vi "Rename State.vi"(8 "error in":errorcluster, 9 "new state":string, 10 "state":string, 11 "routing channel in":T1 format="%.0x") -> (0 "error out":errorcluster, 3 "routing channel out":T1=18446744073709551615 format="%.0x")   [LabVIEW 2020, in "Routing and Faulting Scripting.lvlib"]
doc: "Changes the name of an existing state."
uses:
  Routing and Faulting Scripting.lvlib
  <vilib>/NI VeriStand/Custom Device API/Custom Device Item Ref.ctl
  <vilib>/NI VeriStand/Custom Device API/Custom Device API.lvlib
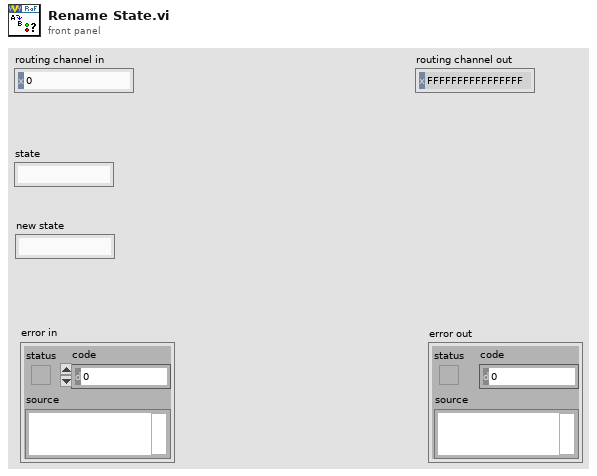
[diagram p1: front panel]
types:
  T1 = typedef "Custom Device API.lvlib/Custom Device Item Ref.ctl" = u64
  T2 = typedef "Routing and Faulting Shared.lvlib/Channel States.ctl" = T3[]
  T3 = typedef "Routing and Faulting Shared.lvlib/Routing State.ctl" = cluster{"Name":string, "Description":string, "Value":i32, "Connection List":T4[]}
  T4 = typedef "Routing and Faulting Shared.lvlib/Connection.ctl" = cluster{"Module":string, "Source":string, "Destination":string}
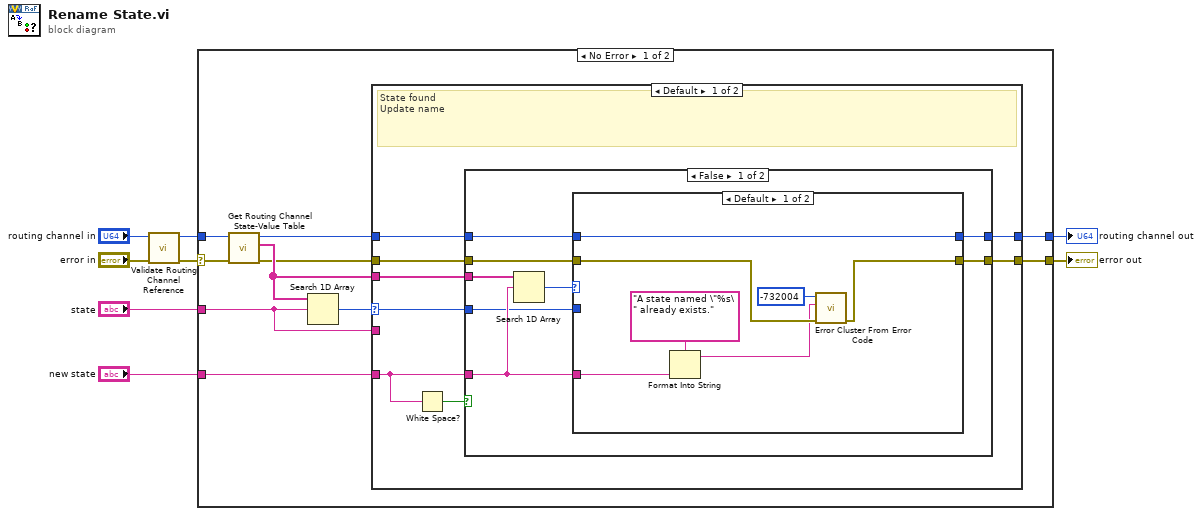
[diagram p0: block diagram]
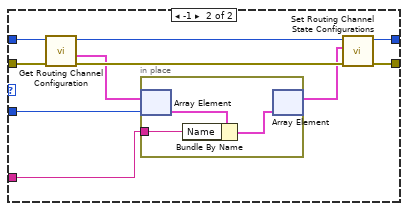
[diagram p2: hidden frame]
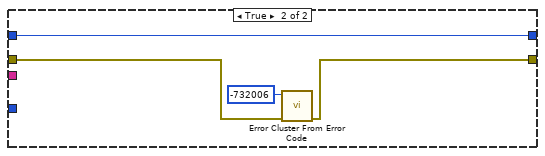
[diagram p3: hidden frame]
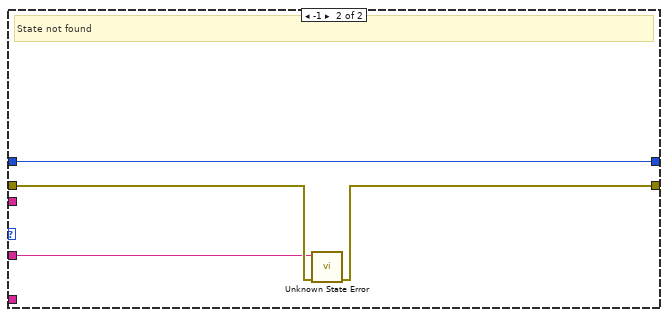
[diagram p4: hidden frame]
diagram:
  n1 = call "Validate Routing Channel Reference.vi"("error in"="error in", "routing channel in"="routing channel in") -> ("error out"=w3:errorcluster, "routing channel out"=w1:T1)  [unwired: 8 in]
  n2 = case shown="No Error" w3 {
    selector: w3 -> [w17 w64]
    tunnel: [w14 w64] -> w5
    tunnel: w1 -> [w18 w63]
    tunnel: [w15 w63] -> w7
    tunnel: "state" -> [w10 _]
    tunnel: "new state" -> [w12 _]
    frame No Error {
      n3 = call "Get Routing Channel State-Value Table.vi"("error in"=w17, "routing channel in"=w18) -> ("error out"=w9:errorcluster, "state names"=w13:string[], "routing channel out"=w16:T1)  [unwired: 6 in, 1 out]
      n4 = Search 1D Array(1D array=w13, element=w10) -> (index of element=w11:i32)  [unwired: 1 in]
      n5 = case shown="Default" w11 {
        selector: w11 -> [w21 _]
        tunnel: w16 -> [w26 w60]
        tunnel: w9 -> [w25 w62]
        tunnel: [w22 w60] -> w15
        tunnel: [w23 w61] -> w14
        tunnel: w12 -> [w20 _]
        tunnel: w13 -> [w24 _]
        tunnel: w10 -> [_ w59]
        frame Default {
          # "State found\nUpdate name"
          n6 = White Space?(1:w20) -> (0:w19:bool)
          n7 = case shown="False" w19 {
            tunnel: w26 -> [w34 w57]
            tunnel: w25 -> [w33 w56]
            tunnel: w24 -> [w32 _]
            tunnel: w20 -> [w31 _]
            tunnel: [w30 w55] -> w23
            tunnel: [w28 w57] -> w22
            tunnel: w21 -> [w27 _]
            frame False {
              n8 = Search 1D Array(1D array=w32, element=w31) -> (index of element=w29:i32)  [unwired: 1 in]
              n9 = case shown="Default" w29 {
                tunnel: w34 -> [w39 w49]
                tunnel: w33 -> [w40 w42]
                tunnel: w31 -> [w36 w48]
                tunnel: [w38 w43] -> w30
                tunnel: [w39 w44] -> w28
                tunnel: w27 -> [_ w47]
                frame Default {
                  n10 = Format Into String(format string="A state named \"%s\" already exists." ("error message (\"\")"), w36) -> (resulting string=w35:string)  [unwired: 2 in, 1 out]
                  n11 = call <vilib>:"Error Cluster From Error Code.vi"("error in (no error)"=w40, "error message (\"\")"=w35, "error code (0)"=-732004) -> ("error out"=w38:errorcluster)  [unwired: 6 in]
                }
                frame -1 {
                  n12 = call "Get Routing Channel Configuration.vi"("error in"=w42, "routing channel in"=w49) -> ("error out"=w50:errorcluster, "state configurations"=w46:T2, "routing channel out"=w51:T1)  [unwired: 4 in, 3 out]
                  n13 = in-place {
                    in-place-border: w48 -> [w54]
                    n14 = in-place-array #1(w46, w47) -> (w53:T3)
                    n15 = Bundle By Name(cluster=w53, "Name"=w54) -> (w52:T3)
                    n16 = in-place-array #1(w52) -> (w45:T2)  [unwired: 1 out]
                  }
                  n17 = call "Set Routing Channel State Configurations.vi"("error in"=w50, "state configurations"=w45, "routing channel in"=w51) -> ("error out"=w43:errorcluster, "routing channel out"=w44:T1)  [unwired: 7 in]
                }
              }
            }
            frame True {
              n18 = call <vilib>:"Error Cluster From Error Code.vi"("error in (no error)"=w56, "error code (0)"=-732006) -> ("error out"=w55:errorcluster)  [unwired: 7 in]
            }
          }
        }
        frame -1 {
          # "State not found"
          n19 = call "Unknown State Error.vi"("error in (no error)"=w62, "state"=w59) -> ("error out"=w61:errorcluster)  [unwired: 9 in]
        }
      }
    }
    frame Error {
    }
  }
  "routing channel out" <- w7
  "error out" <- w5
